vi "Get Service Settings.vi"(8 "error in (no error)":errorcluster) -> (0 "error out":errorcluster, 3 "service settings":T1)   [LabVIEW 2021, in "AudioGenUtility.lvlib"]
uses:
  AudioGenUtility.lvlib
  controls/service settings.ctl
  controls/AudioGenTypeDefs.lvlib
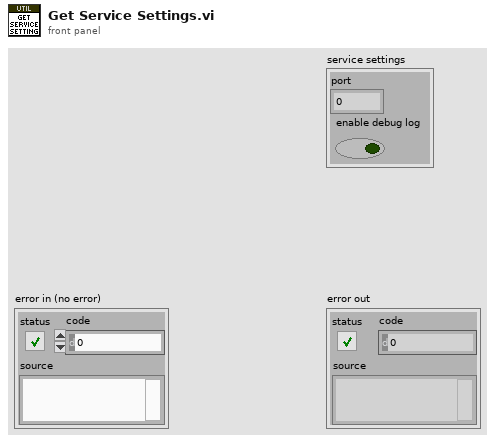
[diagram p1: front panel]
types:
  T1 = typedef "AudioGenTypeDefs.lvlib/service settings.ctl" = cluster{"port":u32, "enable debug log":bool}
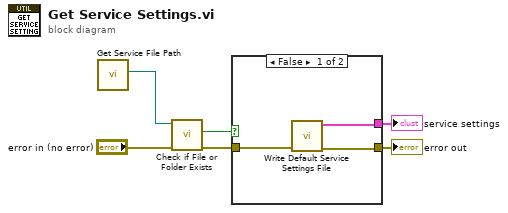
[diagram p0: block diagram]
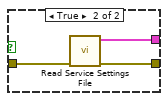
[diagram p2: hidden frame]
diagram:
  n1 = call "Get Service File Path.vi"() -> ("service setting file"=w5:path)  [unwired: 11 in]
  n2 = call <vilib>:"Check if File or Folder Exists.vi"("error in (no error)"="error in (no error)", "path"=w5) -> ("error out"=w4:errorcluster, "file or folder exists?"=w3:bool)  [unwired: 7 in, 1 out]
  n3 = case shown="False" w3 {
    tunnel: w4 -> [w9 w12]
    tunnel: [w8 w11] -> w2
    tunnel: [w7 w10] -> w1
    frame False {
      n4 = call "Write Default Service Settings File.vi"("error in (no error)"=w9) -> ("error out"=w8:errorcluster, "service settings"=w7:T1)  [unwired: 9 in]
    }
    frame True {
      n5 = call "Read Service Settings File.vi"("error in (no error)"=w12) -> ("error out"=w11:errorcluster, "service settings"=w10:T1)  [unwired: 9 in]
    }
  }
  "error out" <- w2
  "service settings" <- w1
